vi "WirebirdLabs-Time-Timer.vi"(0 "Previous Time":u32, 11 "error in":errorcluster) -> (4 "Timer (msec)":u32, 6 "Time to Execute (msec)":u32, 8 "Execution Time (msec)":string, 10 "Execution Time (min)":string, 15 "error out":errorcluster)   [LabVIEW 2012]
panel:
  # "Inputs"
  # "Outputs"
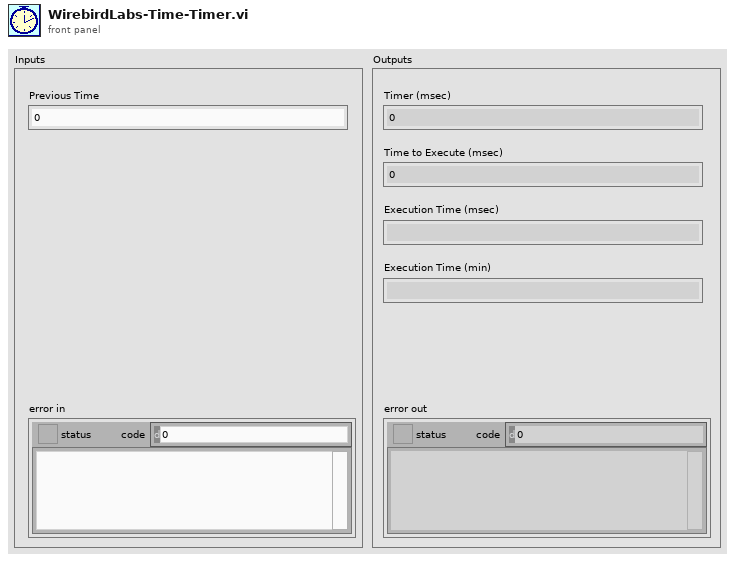
[diagram p1: front panel]
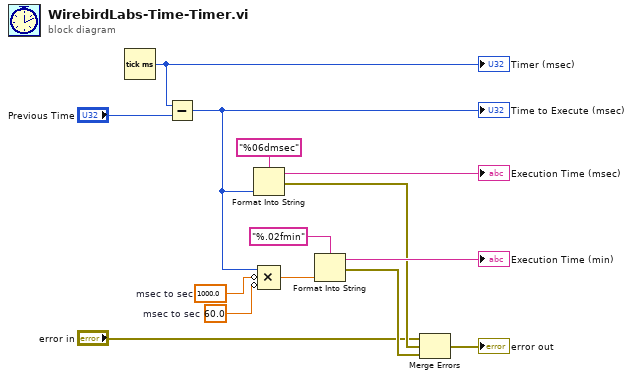
[diagram p0: block diagram]
diagram:
  w9 = 60.0  # msec to sec
  w10 = 1000.0  # msec to sec
  n1 = Tick Count (ms)() -> (millisecond timer value=w14:u32)
  "Timer (msec)" <- w14
  n2 = Subtract(x=w14, y="Previous Time") -> (x-y=w6:u32)
  "Time to Execute (msec)" <- w6
  n3 = Format Into String(format string="%06dmsec", w6) -> (resulting string=→"Execution Time (msec)":string, error out=w4:errorcluster)  [unwired: 2 in]
  n4 = Compound Arithmetic op=MULTIPLY(w6, invert w10, invert w9) -> (w8:dbl)
  n5 = Format Into String(format string="%.02fmin", w8) -> (resulting string=→"Execution Time (min)":string, error out=w3:errorcluster)  [unwired: 2 in]
  n6 = Merge Errors("error in", w4, w3) -> (→"error out":errorcluster)
